vi "TSM SSC DAQmx Stop.vi"(0 "TSM DAQmx In":T1, 11 "error in (no error)":errorcluster) -> (4 "TSM DAQmx Out":T1, 15 "error out":errorcluster)   [LabVIEW 2020]
doc: "Stops the tasks running on DAQmx."
uses:
  Pin Map/TSM DAQmx Multi-Task.ctl
  <vilib>/NI_TestStand_SemiconductorModule/NI_TestStand_Semiconductor_Module.lvlibp/PinMap/PinQueryContext/MultiplePinMultipleSessionQueryContext/MultiplePinMultipleSessionQueryContext.lvclass
  Pin Map/SSC DAQmx.ctl
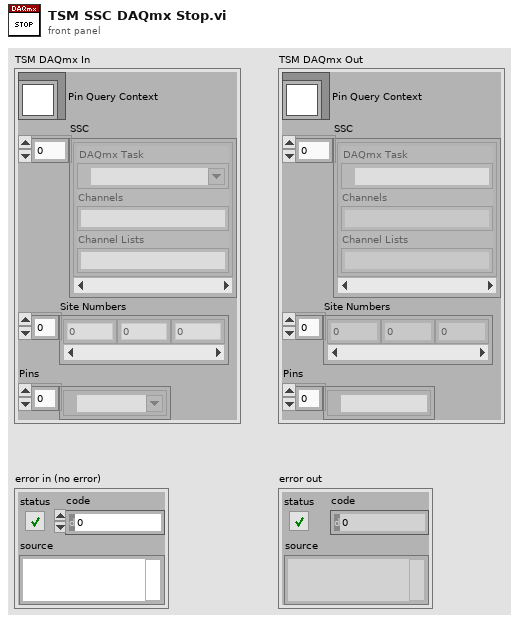
[diagram p1: front panel]
types:
  T1 = typedef "TSM DAQmx Multi-Task.ctl" = cluster{"Pin Query Context":refnum<class "MultiplePinMultipleSessionQueryContext.lvclass">, "SSC":T2[], "Site Numbers":i32[], "Pins":tag[]}
  T2 = typedef "SSC DAQmx.ctl" = cluster{"DAQmx Task ":refnum<k21>, "Channels":string, "Channel Lists":string}
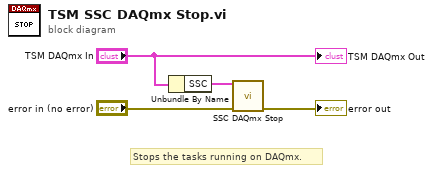
[diagram p0: block diagram]
diagram:
  # "Stops the tasks running on DAQmx."
  n1 = Unbundle By Name("TSM DAQmx In") -> ("SSC"=w1:T2[])
  n2 = call "SSC DAQmx Stop.vi"("DAQmx SSC in"=w1, "error in"="error in (no error)") -> ("error out"=→"error out":errorcluster)  [unwired: 12 in, 1 out]
  "TSM DAQmx Out" <- "TSM DAQmx In"
